vi "Z_Q_4952.vi"(9 "Type":string) -> (0 "Qn":dbl[](array[numeric]), 2 "L":i32)   [LabVIEW 2019]
panel:
  in  "External Qn":dbl[](array[numeric])
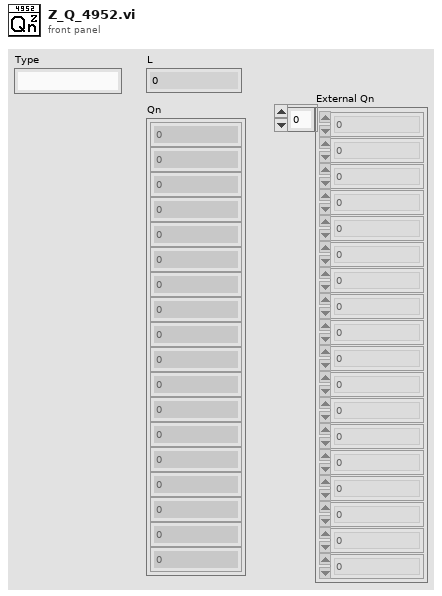
[diagram p1: front panel]
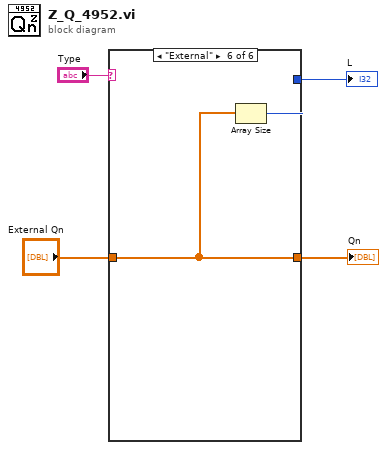
[diagram p0: block diagram]
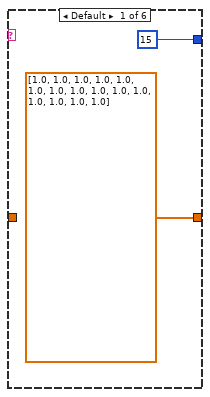
[diagram p2: hidden frame]
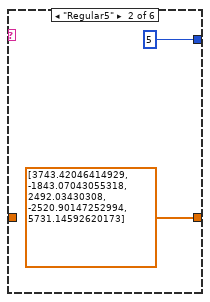
[diagram p3: hidden frame]
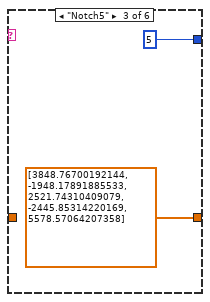
[diagram p4: hidden frame]
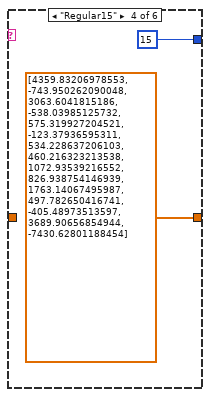
[diagram p5: hidden frame]
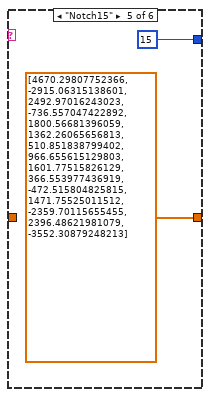
[diagram p6: hidden frame]
diagram:
  n1 = case shown="\"External\"" "Type" {
    tunnel: [15 5 5 15 15 w15] -> w3
    tunnel: [dbl[] [1.0, 1.0, 1.0, 1.0, 1.0, 1.0, 1.0, 1.0, 1.0, 1.0, 1.0, 1.0, 1.0, 1.0, 1.0] ("Qn") dbl[] [3743.42046414929, -1843.07043055318, 2492.03430308, -2520.90147252994, 5731.14592620173] ("Qn") dbl[] [3848.76700192144, -1948.17891885533, 2521.74310409079, -2445.85314220169, 5578.57064207358] ("Qn") dbl[] [4359.83206978553, -743.950262090048, 3063.6041815186, -538.03985125732, 575.319927204521, -123.37936595311, 534.228637206103, 460.216323213538, 1072.93539216552, 826.938754146939, 1763.14067495987, 497.782650416741, -405.48973513597, 3689.90656854944, -7430.62801188454] ("Qn") dbl[] [4670.29807752366, -2915.06315138601, 2492.97016243023, -736.557047422892, 1800.56681396059, 1362.26065656813, 510.851838799402, 966.655615129803, 1601.77515826129, 366.553977436919, -472.515804825815, 1471.75525011512, -2359.70115655455, 2396.48621981079, -3552.30879248213] ("Qn") w16] -> w1
    tunnel: "External Qn" -> [_ _ _ _ _ w16]
    frame Default {
    }
    frame "Regular5" {
    }
    frame "Notch5" {
    }
    frame "Regular15" {
    }
    frame "Notch15" {
    }
    frame "External" {
      n2 = Array Size(array=w16) -> (size(s)=w15:i32)
    }
  }
  "Qn" <- w1
  "L" <- w3
